vi "Initialize FP.vi"(5 "Wash Options Ref":refnum<vi>, 7 "Wash Entry Ref":refnum<vi>, 8 "error in":errorcluster, 9 "Enable\\Disable Wash Options":T1(ring), 10 "Wash In Progress Color":cluster{u32, u32}[](array[cluster])=[{6618880, 6618880}], 11 "Wash In Progress Text":string) -> (0 "error out":errorcluster)   [LabVIEW 2020]
doc: "Initialize Front Panel: Wash Entry text/color and Wash options enable status."
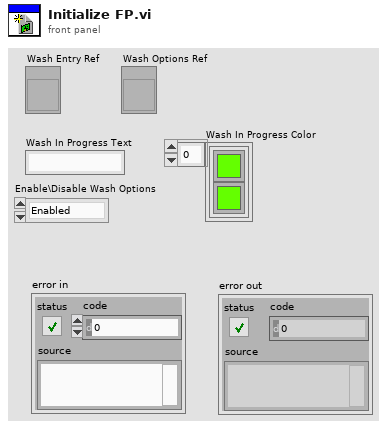
[diagram p1: front panel]
types:
  T1 = enum8{"Enabled", "Disabled", "Disabled and Grayed Out"}
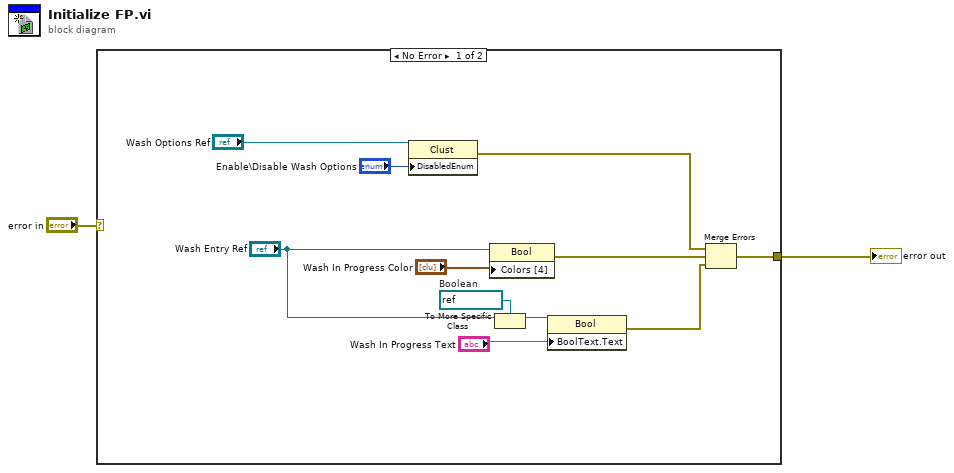
[diagram p0: block diagram]
diagram:
  n1 = case shown="No Error" "error in" {
    selector: "error in" -> [_ w14]
    tunnel: [w7 w14] -> w2
    frame No Error {
      w11 = refnum<vi> refnum  # Boolean
      n2 = property class="Clust"(reference="Wash Options Ref", "DisabledEnum"="Enable\\Disable Wash Options") -> (error out=w5:errorcluster)  [unwired: 1 in, 1 out]
      n3 = property class="Bool"(reference="Wash Entry Ref", "Colors [4]"="Wash In Progress Color") -> (error out=w4:errorcluster)  [unwired: 1 in, 1 out]
      n4 = To More Specific Class(target class=w11, reference="Wash Entry Ref") -> (specific class reference=w12:refnum<vi>)  [unwired: 1 in, 1 out]
      n5 = property class="Bool"(reference=w12, "BoolText.Text"="Wash In Progress Text") -> (error out=w3:errorcluster)  [unwired: 1 in, 1 out]
      n6 = Merge Errors(w5, w4, w3) -> (w7:errorcluster)
    }
    frame Error {
    }
  }
  "error out" <- w2
